vi "RS232发送接收.vi"() -> ()   [LabVIEW 2010]
uses:
  <vilib>/Instr/_visa.llb/VISA Configure Serial Port (Instr).vi
panel:
  out "接收数据_2 2":string
  out "成功_2？ 2":bool caption="成功？"
  in  "发送数据_2 2":string
  out "接收数据_2":string
  out "成功_2？":bool caption="成功？"
  in  "发送数据_2":string
  in  "btn_关闭":bool
  in  "btn_开始测试":bool
  out "接收数据_1":string
  out "成功_1？":bool caption="成功？"
  in  "发送数据_1":string
  # "RS232测试界面"
  # "1#发送字符"
  # "2#发送字符"
  # "1#接收字符"
  # "2#接收字符"
  # "1#测试结果"
  # "2#测试结果"
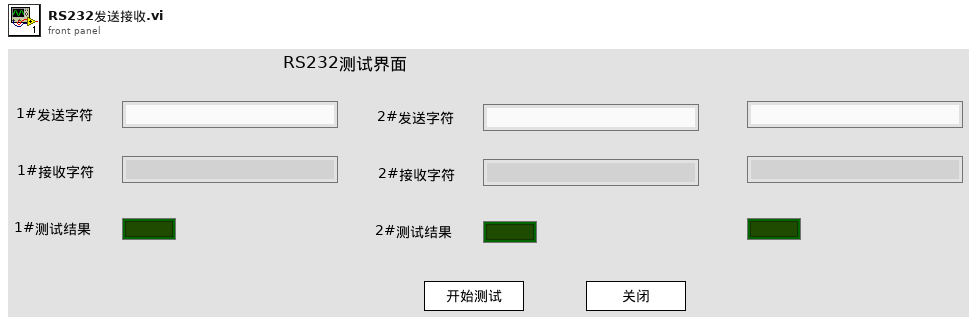
[diagram p1: front panel]
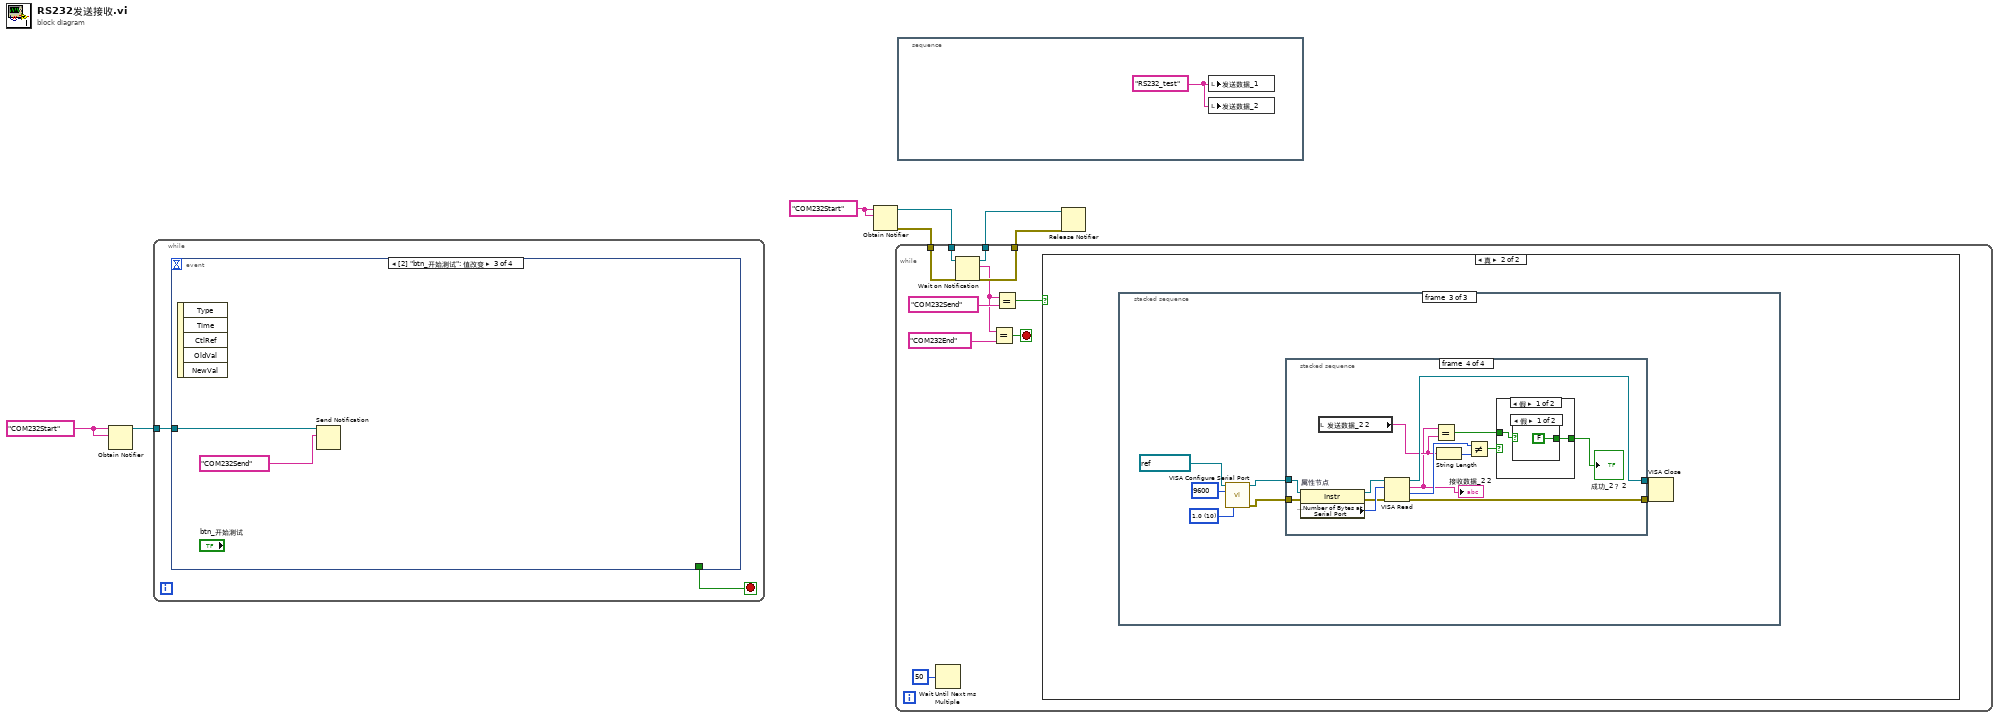
[diagram p0: block diagram]
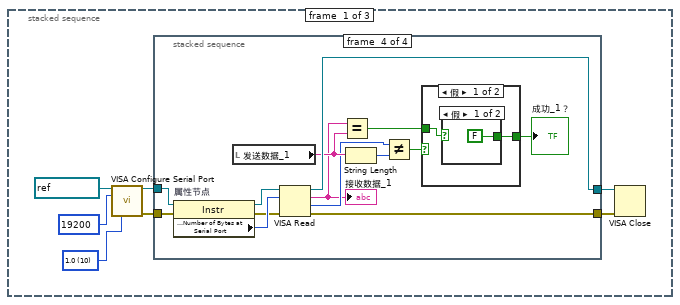
[diagram p3: hidden frame]
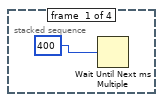
[diagram p4: hidden frame]
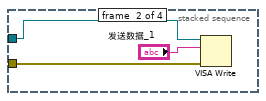
[diagram p5: hidden frame]
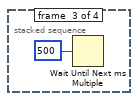
[diagram p6: hidden frame]
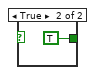
[diagram p7: hidden frame]
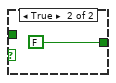
[diagram p8: hidden frame]
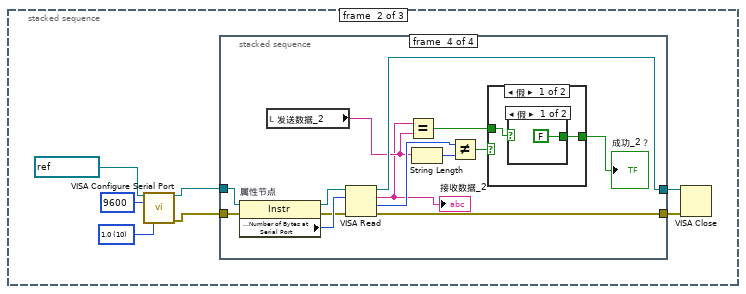
[diagram p9: hidden frame]
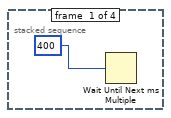
[diagram p10: hidden frame]
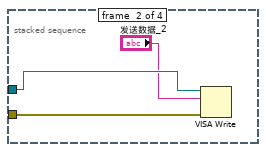
[diagram p11: hidden frame]
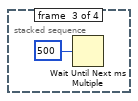
[diagram p12: hidden frame]
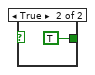
[diagram p13: hidden frame]
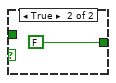
[diagram p14: hidden frame]
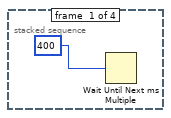
[diagram p15: hidden frame]
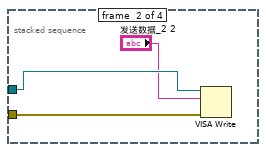
[diagram p16: hidden frame]
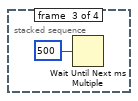
[diagram p17: hidden frame]
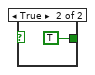
[diagram p18: hidden frame]
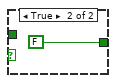
[diagram p19: hidden frame]
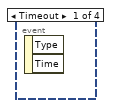
[diagram p20: hidden frame]
diagram:
  w2 = "COM232Start" ("名称（未命名）")
  w7 = "COM232Start" ("名称（未命名）")
  n1 = Obtain Notifier(name (unnamed)=w2, notification data type=w2) -> (notifier out=w1:refnum<notifier>)  [unwired: 2 in, 2 out]
  n2 = while {
    tunnel: w1 -> [w8]
    stop <- w9 stop-if-true
    n3 = event shown="[2] \"btn_开始测试\": 值改变" {
      selector: _ -> [_ _ _ _]
      dyn-events: _ -> [_ _ _ _]
      timeout: _ -> [_ _ _ _]
      tunnel: [_ TRUE _ TRUE] -> w9
      tunnel: w8 -> [_ w11 w13 w15]
      event Timeout {
        n4 = event-data() -> ()  [unwired: 1 in, 2 out]
      }
      event Panel Close {
        n5 = event-data() -> ()  [unwired: 1 in, 3 out]
        n6 = Send Notification(notification="COM232End" ("通知"), notifier=w11) -> ()  [unwired: 1 in, 2 out]
      }
      event "btn_开始测试": Value Change {
        n7 = event-data() -> ()  [unwired: 1 in, 5 out]
        n8 = Send Notification(notification="COM232Send" ("通知"), notifier=w13) -> ()  [unwired: 1 in, 2 out]
      }
      event "btn_关闭": Value Change {
        n9 = event-data() -> ()  [unwired: 1 in, 5 out]
        n10 = Send Notification(notification="COM232End" ("通知"), notifier=w15) -> ()  [unwired: 1 in, 2 out]
      }
    }
  }
  n11 = Obtain Notifier(name (unnamed)=w7, notification data type=w7) -> (notifier out=w6:refnum<notifier>, error out=w5:errorcluster)  [unwired: 2 in, 1 out]
  n12 = while {
    tunnel: w6 -> [w27]
    tunnel: w5 -> [w26]
    tunnel: [w25] -> w4
    tunnel: [w24] -> w3
    stop <- w19 stop-if-true
    n13 = Wait Until Next ms Multiple(millisecond multiple=u32 50 ("毫秒倍数")) -> ()  [unwired: 1 out]
    n14 = Wait on Notification(notifier=w27, error in (no error)=w26) -> (notifier out=w25:refnum<notifier>, notification=w21:string, error out=w24:errorcluster)  [unwired: 2 in, 1 out]
    n15 = Equal?(x=w21, y="COM232End" ("通知")) -> (x = y?=w19:bool)
    n16 = Equal?(x=w21, y="COM232Send" ("通知")) -> (x = y?=w22:bool)
    n17 = case shown="真" w22 {
      frame False {
      }
      frame True {
        n18 = stacked-sequence {
          frame #0 {
            w32 = u16 10 items=["1.0"=10, "1.5"=15, "2.0"=20] ("stop bits (10: 1 bit)")
            n19 = call-poly "VISA Configure Serial Port"("VISA resource name"=refnum<visa-resource-name> "COM1" ("R232端口"), "baud rate (9600)"=u32 19200, "stop bits (10: 1 bit)"=w32) -> ("VISA resource name out"=w31:refnum<visa-resource-name>, "error out"=w30:errorcluster)  [unwired: 11 in]
            n20 = stacked-sequence {
              tunnel: w31 -> [_ w38 _ w51]
              tunnel: w30 -> [_ w37 _ w50]
              tunnel: [_ _ _ w53] -> w29
              tunnel: [_ _ _ w52] -> w28
              frame #0 {
                n21 = Wait Until Next ms Multiple(millisecond multiple=u32 400 ("毫秒倍数")) -> ()  [unwired: 1 out]
              }
              frame #1 {
                n22 = VISA Write(VISA resource name=w38, write buffer="发送数据_1", error in (no error)=w37) -> ()  [unwired: 3 out]
              }
              frame #2 {
                n23 = Wait Until Next ms Multiple(millisecond multiple=u32 500 ("毫秒倍数")) -> ()  [unwired: 1 out]
              }
              frame #3 {
                n24 = property on="属性节点" class="Instr"(reference=w51, error in=w50) -> (reference out=w47:refnum<visa-resource-name>, error out=w45:errorcluster, "Serial Settings:Number of Bytes at Serial Port"=w46:u32)
                n25 = local read "发送数据_1"() -> (w44:string)
                n26 = VISA Read(VISA resource name=w47, byte count=w46, error in (no error)=w45) -> (VISA resource name out=w53:refnum<visa-resource-name>, read buffer=w40:string, return count=w43:u32, error out=w52:errorcluster)
                "接收数据_1" <- w40
                n27 = Equal?(x=w40, y=w44) -> (x = y?=w49:bool)
                n28 = String Length(string=w44) -> (length=w42:i32)
                n29 = Not Equal?(x=w43, y=w42) -> (x != y?=w41:bool)
                n30 = case shown="假" w41 {
                  tunnel: w49 -> [w55 _]
                  tunnel: [w54 FALSE] -> w48
                  frame False {
                    n31 = case shown="假" w55 {
                      tunnel: [FALSE TRUE] -> w54
                      frame False {
                      }
                      frame True {
                      }
                    }
                  }
                  frame True {
                  }
                }
                "成功_1？" <- w48
              }
            }
            n32 = VISA Close(VISA resource name=w29, error in (no error)=w28) -> ()  [unwired: 1 out]
          }
          frame #1 {
            w63 = u16 10 items=["1.0"=10, "1.5"=15, "2.0"=20] ("stop bits (10: 1 bit)")
            n33 = call-poly "VISA Configure Serial Port"("VISA resource name"=refnum<visa-resource-name> "COM3" ("R232端口"), "baud rate (9600)"=u32 9600, "stop bits (10: 1 bit)"=w63) -> ("VISA resource name out"=w60:refnum<visa-resource-name>, "error out"=w59:errorcluster)  [unwired: 11 in]
            n34 = stacked-sequence {
              tunnel: w60 -> [_ w69 _ w82]
              tunnel: w59 -> [_ w68 _ w81]
              tunnel: [_ _ _ w84] -> w65
              tunnel: [_ _ _ w83] -> w64
              frame #0 {
                n35 = Wait Until Next ms Multiple(millisecond multiple=u32 400 ("毫秒倍数")) -> ()  [unwired: 1 out]
              }
              frame #1 {
                n36 = VISA Write(VISA resource name=w69, write buffer="发送数据_2", error in (no error)=w68) -> ()  [unwired: 3 out]
              }
              frame #2 {
                n37 = Wait Until Next ms Multiple(millisecond multiple=u32 500 ("毫秒倍数")) -> ()  [unwired: 1 out]
              }
              frame #3 {
                n38 = property on="属性节点" class="Instr"(reference=w82, error in=w81) -> (reference out=w79:refnum<visa-resource-name>, error out=w77:errorcluster, "Serial Settings:Number of Bytes at Serial Port"=w78:u32)
                n39 = local read "发送数据_2"() -> (w73:string)
                n40 = VISA Read(VISA resource name=w79, byte count=w78, error in (no error)=w77) -> (VISA resource name out=w84:refnum<visa-resource-name>, read buffer=w72:string, return count=w76:u32, error out=w83:errorcluster)
                "接收数据_2" <- w72
                n41 = Equal?(x=w72, y=w73) -> (x = y?=w80:bool)
                n42 = String Length(string=w73) -> (length=w75:i32)
                n43 = Not Equal?(x=w76, y=w75) -> (x != y?=w74:bool)
                n44 = case shown="假" w74 {
                  tunnel: w80 -> [w86 _]
                  tunnel: [w85 FALSE] -> w71
                  frame False {
                    n45 = case shown="假" w86 {
                      tunnel: [FALSE TRUE] -> w85
                      frame False {
                      }
                      frame True {
                      }
                    }
                  }
                  frame True {
                  }
                }
                "成功_2？" <- w71
              }
            }
            n46 = VISA Close(VISA resource name=w65, error in (no error)=w64) -> ()  [unwired: 1 out]
          }
          frame #2 {
            w94 = u16 10 items=["1.0"=10, "1.5"=15, "2.0"=20] ("stop bits (10: 1 bit)")
            n47 = call-poly "VISA Configure Serial Port"("VISA resource name"=refnum<visa-resource-name> "COM4" ("R232端口"), "baud rate (9600)"=u32 9600, "stop bits (10: 1 bit)"=w94) -> ("VISA resource name out"=w91:refnum<visa-resource-name>, "error out"=w90:errorcluster)  [unwired: 11 in]
            n48 = stacked-sequence {
              tunnel: w91 -> [_ w100 _ w113]
              tunnel: w90 -> [_ w99 _ w112]
              tunnel: [_ _ _ w115] -> w96
              tunnel: [_ _ _ w114] -> w95
              frame #0 {
                n49 = Wait Until Next ms Multiple(millisecond multiple=u32 400 ("毫秒倍数")) -> ()  [unwired: 1 out]
              }
              frame #1 {
                n50 = VISA Write(VISA resource name=w100, write buffer="发送数据_2 2", error in (no error)=w99) -> ()  [unwired: 3 out]
              }
              frame #2 {
                n51 = Wait Until Next ms Multiple(millisecond multiple=u32 500 ("毫秒倍数")) -> ()  [unwired: 1 out]
              }
              frame #3 {
                n52 = property on="属性节点" class="Instr"(reference=w113, error in=w112) -> (reference out=w110:refnum<visa-resource-name>, error out=w108:errorcluster, "Serial Settings:Number of Bytes at Serial Port"=w109:u32)
                n53 = local read "发送数据_2 2"() -> (w104:string)
                n54 = VISA Read(VISA resource name=w110, byte count=w109, error in (no error)=w108) -> (VISA resource name out=w115:refnum<visa-resource-name>, read buffer=w103:string, return count=w107:u32, error out=w114:errorcluster)
                "接收数据_2 2" <- w103
                n55 = Equal?(x=w103, y=w104) -> (x = y?=w111:bool)
                n56 = String Length(string=w104) -> (length=w106:i32)
                n57 = Not Equal?(x=w107, y=w106) -> (x != y?=w105:bool)
                n58 = case shown="假" w105 {
                  tunnel: w111 -> [w117 _]
                  tunnel: [w116 FALSE] -> w102
                  frame False {
                    n59 = case shown="假" w117 {
                      tunnel: [FALSE TRUE] -> w116
                      frame False {
                      }
                      frame True {
                      }
                    }
                  }
                  frame True {
                  }
                }
                "成功_2？ 2" <- w102
              }
            }
            n60 = VISA Close(VISA resource name=w96, error in (no error)=w95) -> ()  [unwired: 1 out]
          }
        }
      }
    }
  }
  n61 = stacked-sequence {
    frame #0 {
      w121 = "RS232_test" ("发送数据_1")
      n62 = local write "发送数据_1"(w121) -> ()
      n63 = local write "发送数据_2"(w121) -> ()
    }
  }
  n64 = Release Notifier(notifier=w4, error in (no error)=w3) -> ()  [unwired: 1 in, 3 out]
